vi "Test 10.vi"() -> ()   [LabVIEW 2020]
panel:
  out "Period (msec)":sgl
  out "Period (ticks)":u32
  in  "Speed (RPM)":sgl
  in  "PulsesPerRotation":sgl=60.0 format="%#_6f"
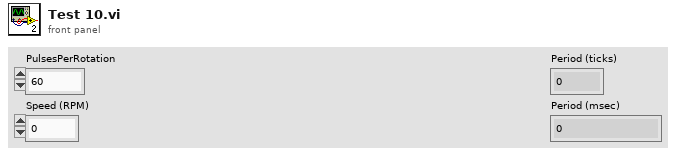
[diagram p1: front panel]
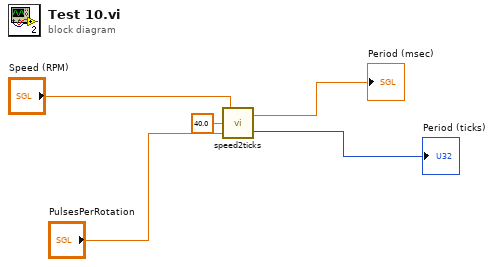
[diagram p0: block diagram]
diagram:
  n1 = call <vilib>:"speed2ticks.vi"("PulsesPerRotation"="PulsesPerRotation", "Clock Frequency (MHz, 40)"=sgl 40.0, "Speed (RPM)"="Speed (RPM)") -> ("Period (ticks)"=→"Period (ticks)":u32, "Period (msec)"=→"Period (msec)":sgl)
